vi "Get Control References.vi"(3 "error in":errorcluster) -> (0 "error out":errorcluster, 1 "Control Reference Cluster":T1)   [LabVIEW 2016]
doc: "Returns an array of control references and a string array of control label names, from the front panel of the calling VI.\n\nThis VI also accounts for tab controls within other tab controls."
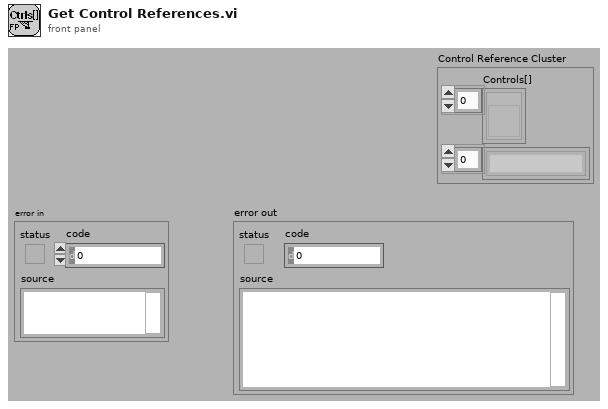
[diagram p1: front panel]
types:
  T1 = cluster{"Controls[]":refnum<vi>[], "Control Names":string[]}
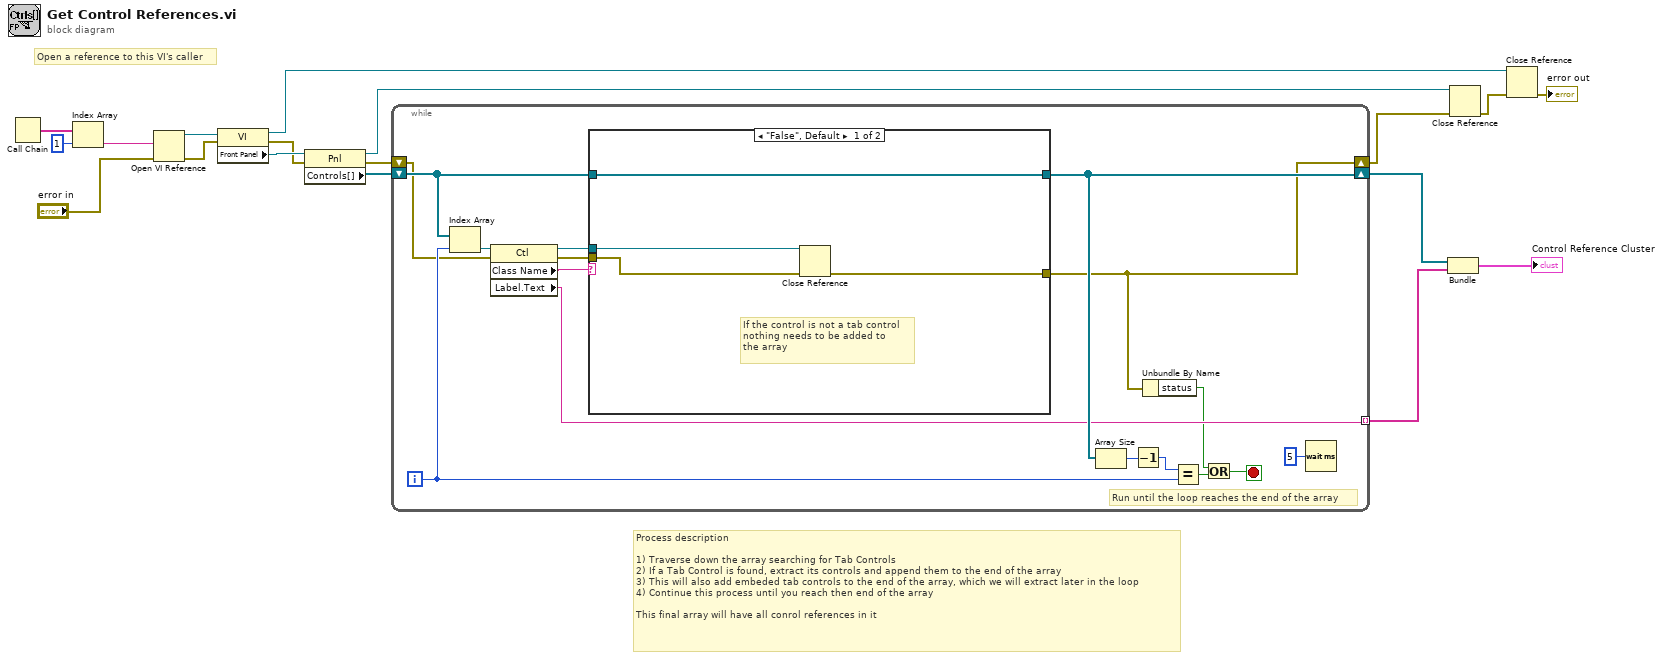
[diagram p0: block diagram]
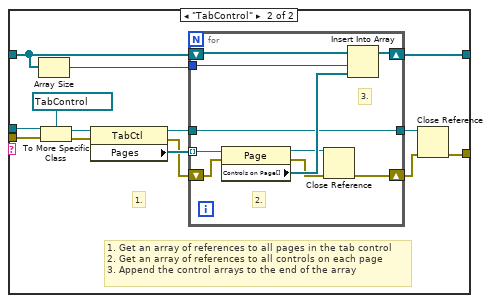
[diagram p2: hidden frame]
diagram:
  # "Open a reference to this VI's caller"
  # "Process description\n\n1) Traverse down the array searching for Tab Controls\n2) If a Tab Control is found, extract its controls and append them to the end of the array\n3) This will also add embeded tab controls to the end of the array, which we will extract later in the loop\n4) Continue this process until you reach then end of the array\n\nThis final array will have all conrol references in it"
  n1 = Call Chain() -> (call chain=w13:string[])
  n2 = Index Array(array=w13, index=1) -> (element=w4:string)
  n3 = Open VI Reference(vi path=w4, error in (no error)="error in") -> (vi reference=w12:refnum<vi>, error out=w11:errorcluster)  [unwired: 4 in]
  n4 = property class="VI"(reference=w12, error in=w11) -> (reference out=w10:refnum<vi>, error out=w16:errorcluster, "Front Panel"=w17:refnum<vi>)
  n5 = property class="Pnl"(reference=w17, error in=w16) -> (reference out=w9:refnum<vi>, error out=w15:errorcluster, "Controls[]"=w18:refnum<vi>[])
  n6 = while {
    shift-right: [w26] -> w3
    shift-left: w18 -> [w32]
    tunnel: [w23] -> w2 mode=indexing
    shift-right: [w22] -> w7
    shift-left: w15 -> [w25]
    i -> [w27]
    stop <- w20 stop-if-true
    # "Run until the loop reaches the end of the array"
    n7 = Index Array(array=w32, index=w27) -> (element=w28:refnum<vi>)
    n8 = property class="Ctl"(reference=w28, error in=w25) -> (reference out=w33:refnum<vi>, error out=w24:errorcluster, "Class Name"=w31:string, "Label.Text"=w23:string)
    n9 = case shown="\"False\", Default" w31 {
      tunnel: w33 -> [w37 w52]
      tunnel: w32 -> [w38 w48]
      tunnel: [w38 w49] -> w26
      tunnel: w24 -> [w36 w45]
      tunnel: [w35 w41] -> w22
      frame "False", Default {
        # "If the control is not a tab control\nnothing needs to be added to\nthe array"
        n10 = Close Reference(reference=w37, error in (no error)=w36) -> (error out=w35:errorcluster)
      }
      frame "TabControl" {
        # "1. Get an array of references to all pages in the tab control\n2. Get an array of references to all controls on each page\n3. Append the control arrays to the end of the array"
        # "1."
        n11 = Array Size(array=w48) -> (size(s)=w46:i32)
        n12 = To More Specific Class(target class=refnum<vi> refnum ("Tab Control"), reference=w52, error in=w45) -> (specific class reference=w51:refnum<vi>, error out=w44:errorcluster)
        n13 = property class="TabCtl"(reference=w51, error in=w44) -> (reference out=w42:refnum<vi>, error out=w43:errorcluster, "Pages"=w50:refnum<vi>[])
        n14 = for {
          tunnel: w50 -> [w62] mode=indexing
          tunnel: w46 -> [w60]
          shift-right: [w61] -> w49
          shift-left: w48 -> [w59]
          tunnel: w42 -> [w56]
          tunnel: [w56] -> w40
          shift-right: [w53] -> w39
          shift-left: w43 -> [w57]
          # "3."
          # "2."
          n15 = property class="Page"(reference=w62, error in=w57) -> (reference out=w55:refnum<vi>, error out=w54:errorcluster, "Controls on Page[]"=w58:refnum<vi>[])
          n16 = Close Reference(reference=w55, error in (no error)=w54) -> (error out=w53:errorcluster)
          n17 = Insert Into Array(array=w59, index=w60, new element=w58) -> (w61:refnum<vi>[])
        }
        n18 = Close Reference(reference=w40, error in (no error)=w39) -> (error out=w41:errorcluster)
      }
    }
    n19 = Array Size(array=w26) -> (size(s)=w30:i32)
    n20 = Decrement(x=w30) -> (x-1=w29:i32)
    n21 = Unbundle By Name(w22) -> ("status"=w19:bool)
    n22 = Equal?(x=w29, y=w27) -> (x = y?=w21:bool)
    n23 = Or(x=w19, y=w21) -> (x .or. y?=w20:bool)
    n24 = Wait (ms)(milliseconds to wait=u32 5) -> ()  [unwired: 1 out]
  }
  n25 = Bundle("Controls[]"=w3, w2) -> (→"Control Reference Cluster":cluster{"Controls[]":refnum<vi>[], string[]})  [unwired: 1 in]
  n26 = Close Reference(reference=w9, error in (no error)=w7) -> (error out=w8:errorcluster)
  n27 = Close Reference(reference=w10, error in (no error)=w8) -> (error out=→"error out":errorcluster)
